vi "AutonSelectTest.vi"() -> ()   [LabVIEW 2017]
uses:
  <vilib>/Utility/miscctls.llb/LVPositionTypeDef.ctl
  <vilib>/Utility/miscctls.llb/LVBoundsTypeDef.ctl
panel:
  out "NumCubes":string
  out "Priority":string
  out "StartPos":string
  in  "stop":bool
  in  "Cross? Button":bool
  in  "Three Cube Button":bool
  in  "Two Cube Button":bool
  in  "One Cube Button":bool
  in  "Switch Button":bool
  in  "Scale Button":bool
  in  "Right Button":bool
  in  "Center Button":bool
  in  "Left Button":bool
  # "Num of\nCubes:"
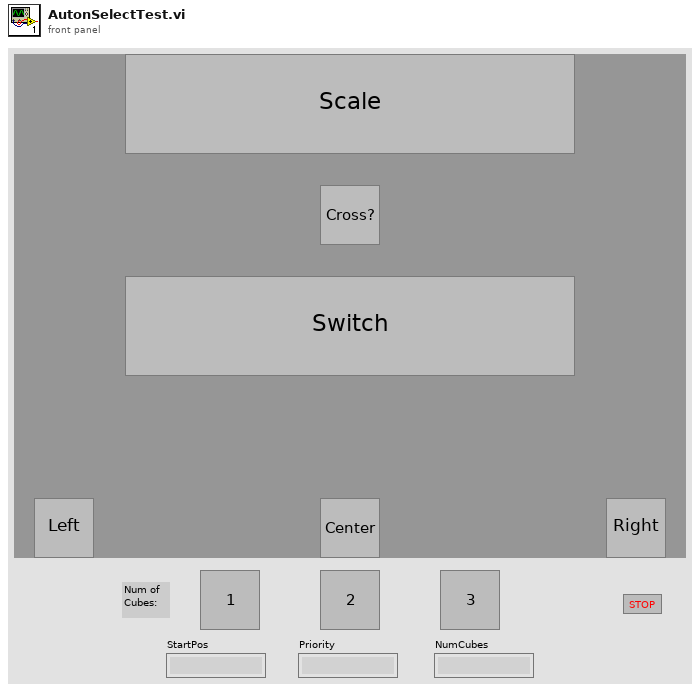
[diagram p1: front panel]
types:
  T1 = typedef "LVPositionTypeDef.ctl" = cluster{"Left":i32, "Top":i32}
  T2 = typedef "LVBoundsTypeDef.ctl" = cluster{"Width":u32, "Height":u32}
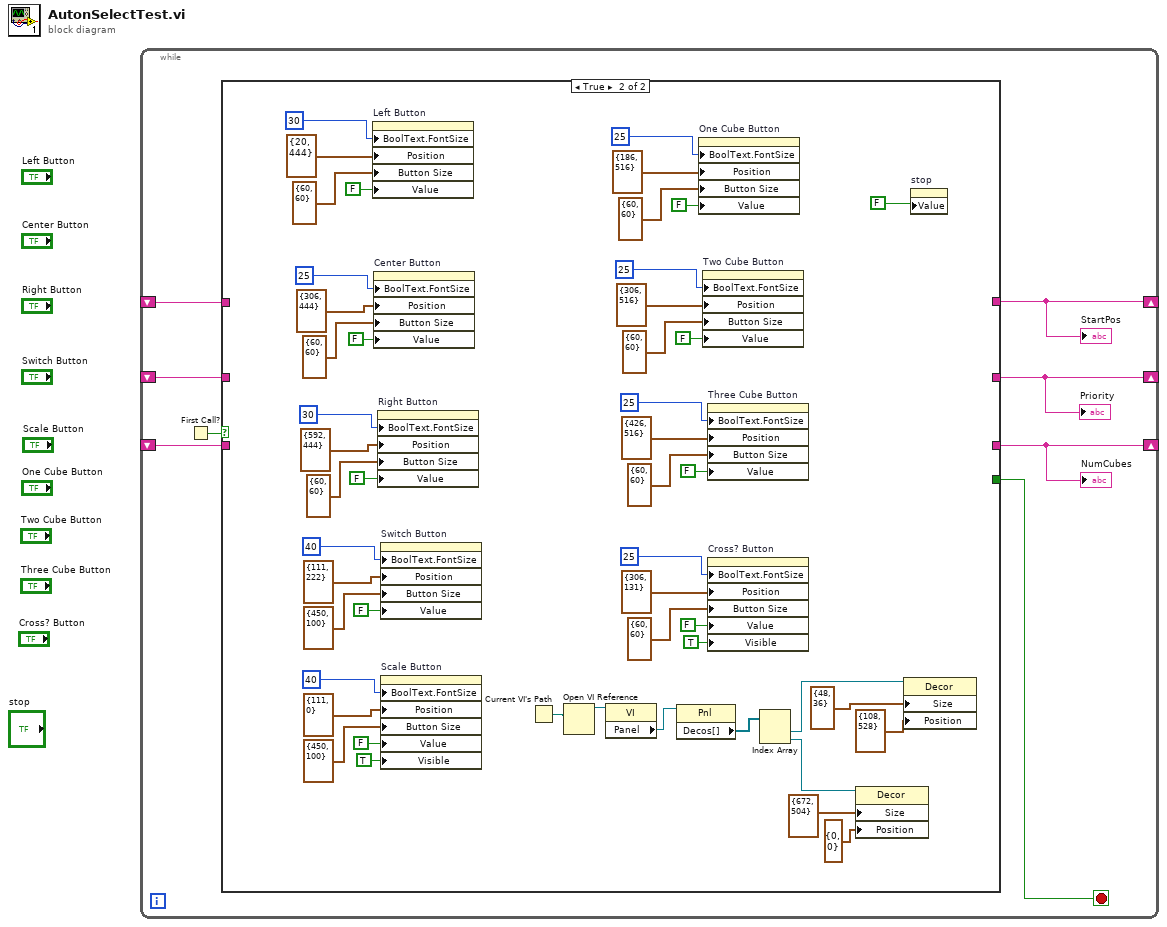
[diagram p0: block diagram]
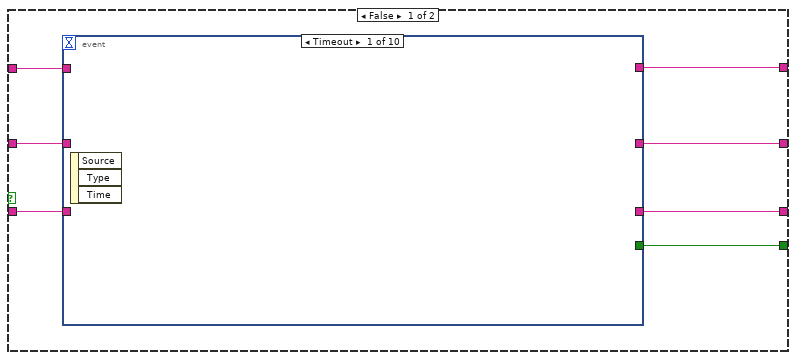
[diagram p2: hidden frame]
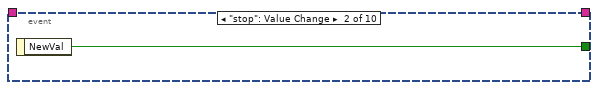
[diagram p3: hidden frame]
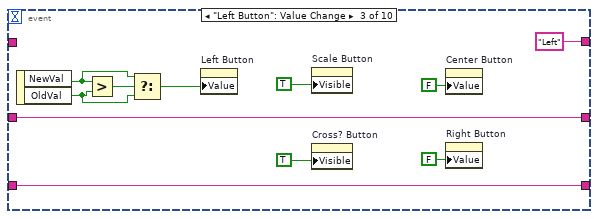
[diagram p4: hidden frame]
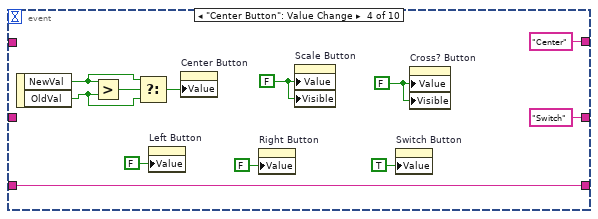
[diagram p5: hidden frame]
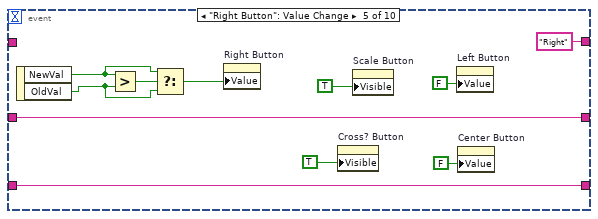
[diagram p6: hidden frame]
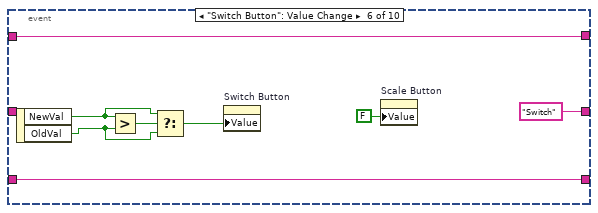
[diagram p7: hidden frame]
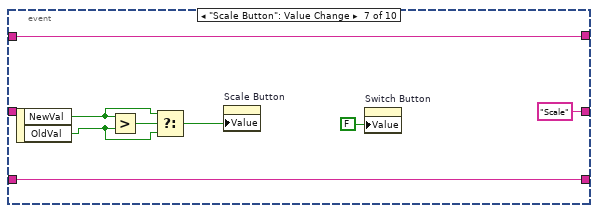
[diagram p8: hidden frame]
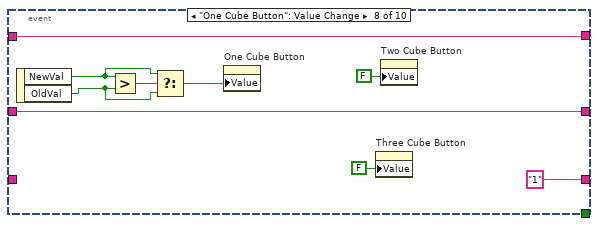
[diagram p9: hidden frame]
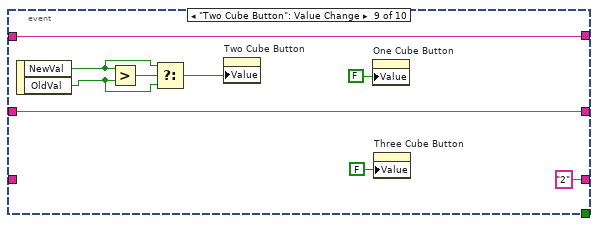
[diagram p10: hidden frame]
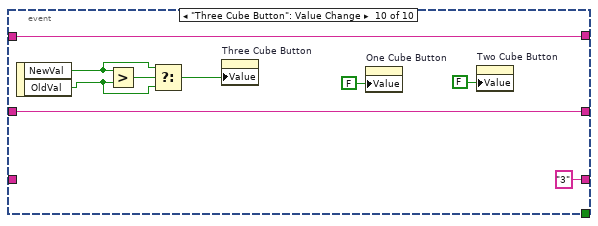
[diagram p11: hidden frame]
diagram:
  n1 = while {
    shift-right: [w4] -> _
    shift-left: _ -> [w3]
    shift-right: [w5] -> _
    shift-left: _ -> [w2]
    shift-right: [w6] -> _
    shift-left: _ -> [w1]
    stop <- w7 stop-if-true
    n2 = First Call?() -> (First Call?: T/F=w8:bool)
    n3 = case shown="True" w8 {
      tunnel: [w15 _] -> w7
      tunnel: [w14 _] -> w4
      tunnel: [w13 _] -> w5
      tunnel: [w12 _] -> w6
      tunnel: w3 -> [w11 _]
      tunnel: w2 -> [w10 _]
      tunnel: w1 -> [w9 _]
      frame False {
        n4 = event shown="[0] Timeout" {
          selector: _ -> [_ _ _ _ _ _ _ _ _ _]
          dyn-events: _ -> [_ _ _ _ _ _ _ _ _ _]
          timeout: _ -> [_ _ _ _ _ _ _ _ _ _]
          tunnel: [_ w16 _ _ _ _ _ _ _ _] -> w15
          tunnel: [_ _ "Left" "Center" "Right" w52 w60 w68 w76 w86] -> w14
          tunnel: [_ _ w18 "Switch" w41 "Switch" "Scale" w67 w77 w85] -> w13
          tunnel: [_ _ w17 w29 w40 w51 w59 "1" "2" "3"] -> w12
          tunnel: w11 -> [_ _ _ _ _ w52 w60 w68 w76 w86]
          tunnel: w10 -> [_ _ w18 _ w41 _ _ w67 w77 w85]
          tunnel: w9 -> [_ _ w17 w29 w40 w51 w59 _ _ _]
          event Timeout {
            n5 = event-data() -> ()  [unwired: 1 in, 3 out]
          }
          event "stop": Value Change {
            n6 = event-data() -> ("NewVal"=w16:bool)  [unwired: 1 in]
          }
          event "Left Button": Value Change {
            n7 = event-data() -> ("NewVal"=w24:bool, "OldVal"=w23:bool)  [unwired: 1 in]
            n8 = Greater?(x=w24, y=w23) -> (0:w25:bool)
            n9 = Select(t=w24, s=w25, f=w23) -> (s? t:f=w22:bool)
            n10 = property on="Left Button" class="Bool (strict)"("Value"=w22) -> ()  [unwired: 2 in, 2 out]
            n11 = property on="Scale Button" class="Bool (strict)"("Visible"=TRUE ("Right Button")) -> ()  [unwired: 2 in, 2 out]
            n12 = property on="Cross? Button" class="Bool (strict)"("Visible"=TRUE ("Right Button")) -> ()  [unwired: 2 in, 2 out]
            n13 = property on="Center Button" class="Bool (strict)"("Value"=FALSE ("Center Button")) -> ()  [unwired: 2 in, 2 out]
            n14 = property on="Right Button" class="Bool (strict)"("Value"=FALSE ("Right Button")) -> ()  [unwired: 2 in, 2 out]
          }
          event "Center Button": Value Change {
            w32 = FALSE ("Right Button")
            w31 = FALSE ("Right Button")
            n15 = event-data() -> ("NewVal"=w34:bool, "OldVal"=w35:bool)  [unwired: 1 in]
            n16 = Greater?(x=w34, y=w35) -> (0:w37:bool)
            n17 = Select(t=w34, s=w37, f=w35) -> (s? t:f=w36:bool)
            n18 = property on="Left Button" class="Bool (strict)"("Value"=FALSE ("Center Button")) -> ()  [unwired: 2 in, 2 out]
            n19 = property on="Center Button" class="Bool (strict)"("Value"=w36) -> ()  [unwired: 2 in, 2 out]
            n20 = property on="Right Button" class="Bool (strict)"("Value"=FALSE ("Right Button")) -> ()  [unwired: 2 in, 2 out]
            n21 = property on="Scale Button" class="Bool (strict)"("Value"=w31, "Visible"=w31) -> ()  [unwired: 2 in, 2 out]
            n22 = property on="Switch Button" class="Bool (strict)"("Value"=TRUE ("Right Button")) -> ()  [unwired: 2 in, 2 out]
            n23 = property on="Cross? Button" class="Bool (strict)"("Value"=w32, "Visible"=w32) -> ()  [unwired: 2 in, 2 out]
          }
          event "Right Button": Value Change {
            n24 = event-data() -> ("NewVal"=w45:bool, "OldVal"=w46:bool)  [unwired: 1 in]
            n25 = Greater?(x=w45, y=w46) -> (0:w48:bool)
            n26 = Select(t=w45, s=w48, f=w46) -> (s? t:f=w47:bool)
            n27 = property on="Right Button" class="Bool (strict)"("Value"=w47) -> ()  [unwired: 2 in, 2 out]
            n28 = property on="Cross? Button" class="Bool (strict)"("Visible"=TRUE ("Right Button")) -> ()  [unwired: 2 in, 2 out]
            n29 = property on="Scale Button" class="Bool (strict)"("Visible"=TRUE ("Right Button")) -> ()  [unwired: 2 in, 2 out]
            n30 = property on="Left Button" class="Bool (strict)"("Value"=FALSE ("Center Button")) -> ()  [unwired: 2 in, 2 out]
            n31 = property on="Center Button" class="Bool (strict)"("Value"=FALSE ("Right Button")) -> ()  [unwired: 2 in, 2 out]
          }
          event "Switch Button": Value Change {
            n32 = event-data() -> ("NewVal"=w54:bool, "OldVal"=w55:bool)  [unwired: 1 in]
            n33 = Greater?(x=w54, y=w55) -> (0:w57:bool)
            n34 = Select(t=w54, s=w57, f=w55) -> (s? t:f=w56:bool)
            n35 = property on="Switch Button" class="Bool (strict)"("Value"=w56) -> ()  [unwired: 2 in, 2 out]
            n36 = property on="Scale Button" class="Bool (strict)"("Value"=FALSE ("Center Button")) -> ()  [unwired: 2 in, 2 out]
          }
          event "Scale Button": Value Change {
            n37 = event-data() -> ("NewVal"=w62:bool, "OldVal"=w63:bool)  [unwired: 1 in]
            n38 = Greater?(x=w62, y=w63) -> (0:w65:bool)
            n39 = Select(t=w62, s=w65, f=w63) -> (s? t:f=w64:bool)
            n40 = property on="Scale Button" class="Bool (strict)"("Value"=w64) -> ()  [unwired: 2 in, 2 out]
            n41 = property on="Switch Button" class="Bool (strict)"("Value"=FALSE ("Center Button")) -> ()  [unwired: 2 in, 2 out]
          }
          event "One Cube Button": Value Change {
            n42 = event-data() -> ("NewVal"=w71:bool, "OldVal"=w72:bool)  [unwired: 1 in]
            n43 = Greater?(x=w71, y=w72) -> (0:w74:bool)
            n44 = Select(t=w71, s=w74, f=w72) -> (s? t:f=w73:bool)
            n45 = property on="One Cube Button" class="Bool (strict)"("Value"=w73) -> ()  [unwired: 2 in, 2 out]
            n46 = property on="Three Cube Button" class="Bool (strict)"("Value"=FALSE ("Center Button")) -> ()  [unwired: 2 in, 2 out]
            n47 = property on="Two Cube Button" class="Bool (strict)"("Value"=FALSE ("Center Button")) -> ()  [unwired: 2 in, 2 out]
          }
          event "Two Cube Button": Value Change {
            n48 = event-data() -> ("NewVal"=w80:bool, "OldVal"=w81:bool)  [unwired: 1 in]
            n49 = Greater?(x=w80, y=w81) -> (0:w83:bool)
            n50 = Select(t=w80, s=w83, f=w81) -> (s? t:f=w82:bool)
            n51 = property on="Two Cube Button" class="Bool (strict)"("Value"=w82) -> ()  [unwired: 2 in, 2 out]
            n52 = property on="One Cube Button" class="Bool (strict)"("Value"=FALSE ("Center Button")) -> ()  [unwired: 2 in, 2 out]
            n53 = property on="Three Cube Button" class="Bool (strict)"("Value"=FALSE ("Center Button")) -> ()  [unwired: 2 in, 2 out]
          }
          event "Three Cube Button": Value Change {
            n54 = event-data() -> ("NewVal"=w89:bool, "OldVal"=w90:bool)  [unwired: 1 in]
            n55 = Greater?(x=w89, y=w90) -> (0:w92:bool)
            n56 = Select(t=w89, s=w92, f=w90) -> (s? t:f=w91:bool)
            n57 = property on="Three Cube Button" class="Bool (strict)"("Value"=w91) -> ()  [unwired: 2 in, 2 out]
            n58 = property on="One Cube Button" class="Bool (strict)"("Value"=FALSE ("Center Button")) -> ()  [unwired: 2 in, 2 out]
            n59 = property on="Two Cube Button" class="Bool (strict)"("Value"=FALSE ("Center Button")) -> ()  [unwired: 2 in, 2 out]
          }
        }
      }
      frame True {
        n60 = property on="Left Button" class="Bool (strict)"("BoolText.FontSize"=u32 30 ("Caption.Font:Size"), "Position"=T1 {"Left"=20, "Top"=444}, "Button Size"=T2 {"Width"=60, "Height"=60}, "Value"=FALSE) -> ()  [unwired: 2 in, 2 out]
        n61 = property on="Center Button" class="Bool (strict)"("BoolText.FontSize"=u32 25 ("Caption.Font:Size"), "Position"=T1 {"Left"=306, "Top"=444}, "Button Size"=T2 {"Width"=60, "Height"=60}, "Value"=FALSE) -> ()  [unwired: 2 in, 2 out]
        n62 = property on="Right Button" class="Bool (strict)"("BoolText.FontSize"=u32 30 ("Caption.Font:Size"), "Position"=T1 {"Left"=592, "Top"=444}, "Button Size"=T2 {"Width"=60, "Height"=60}, "Value"=FALSE) -> ()  [unwired: 2 in, 2 out]
        n63 = property on="Switch Button" class="Bool (strict)"("BoolText.FontSize"=u32 40 ("Caption.Font:Size"), "Position"=T1 {"Left"=111, "Top"=222}, "Button Size"=T2 {"Width"=450, "Height"=100}, "Value"=FALSE) -> ()  [unwired: 2 in, 2 out]
        n64 = property on="Scale Button" class="Bool (strict)"("BoolText.FontSize"=u32 40 ("Caption.Font:Size"), "Position"=T1 {"Left"=111, "Top"=0}, "Button Size"=T2 {"Width"=450, "Height"=100}, "Value"=FALSE, "Visible"=TRUE) -> ()  [unwired: 2 in, 2 out]
        n65 = Current VI's Path() -> (path=w104:path)
        n66 = Open VI Reference(vi path=w104) -> (vi reference=w103:refnum<vi>)  [unwired: 5 in, 1 out]
        n67 = property class="VI"(reference=w103) -> ("Panel"=w102:refnum<vi>)  [unwired: 1 in, 2 out]
        n68 = property class="Pnl"(reference=w102) -> ("Decos[]"=w101:refnum<vi>[])  [unwired: 1 in, 2 out]
        n69 = property on="One Cube Button" class="Bool (strict)"("BoolText.FontSize"=u32 25 ("Caption.Font:Size"), "Position"=T1 {"Left"=186, "Top"=516}, "Button Size"=T2 {"Width"=60, "Height"=60}, "Value"=FALSE) -> ()  [unwired: 2 in, 2 out]
        n70 = property on="Two Cube Button" class="Bool (strict)"("BoolText.FontSize"=u32 25 ("Caption.Font:Size"), "Position"=T1 {"Left"=306, "Top"=516}, "Button Size"=T2 {"Width"=60, "Height"=60}, "Value"=FALSE) -> ()  [unwired: 2 in, 2 out]
        n71 = property on="Three Cube Button" class="Bool (strict)"("BoolText.FontSize"=u32 25 ("Caption.Font:Size"), "Position"=T1 {"Left"=426, "Top"=516}, "Button Size"=T2 {"Width"=60, "Height"=60}, "Value"=FALSE) -> ()  [unwired: 2 in, 2 out]
        n72 = property on="Cross? Button" class="Bool (strict)"("BoolText.FontSize"=u32 25 ("Caption.Font:Size"), "Position"=T1 {"Left"=306, "Top"=131}, "Button Size"=T2 {"Width"=60, "Height"=60}, "Value"=FALSE, "Visible"=TRUE) -> ()  [unwired: 2 in, 2 out]
        n73 = Index Array(array=w101) -> (element #1=w100:refnum<vi>, element #2=w96:refnum<vi>)  [unwired: 2 in]
        n74 = property class="Decor"(reference=w96, "Size"=T2 {"Width"=672, "Height"=504}, "Position"=T1 {"Left"=0, "Top"=0}) -> ()  [unwired: 1 in, 2 out]
        n75 = property class="Decor"(reference=w100, "Size"=T2 {"Width"=48, "Height"=36}, "Position"=T1 {"Left"=108, "Top"=528}) -> ()  [unwired: 1 in, 2 out]
        n76 = property on="stop" class="Bool (strict)"("Value"=FALSE) -> ()  [unwired: 2 in, 2 out]
      }
    }
    "StartPos" <- w4
    "Priority" <- w5
    "NumCubes" <- w6
  }
